vi "controlAutoReset.vi"(7 "Set":bool, 8 "error in":errorcluster, 9 "auto reset in":bool=TRUE, 10 "axis in":u8, 11 "connection ID":i32) -> (0 "error out":errorcluster, 1 "auto reset out":bool=TRUE, 2 "axis out":u8, 3 "connection ID":i32)   [LabVIEW 2016]
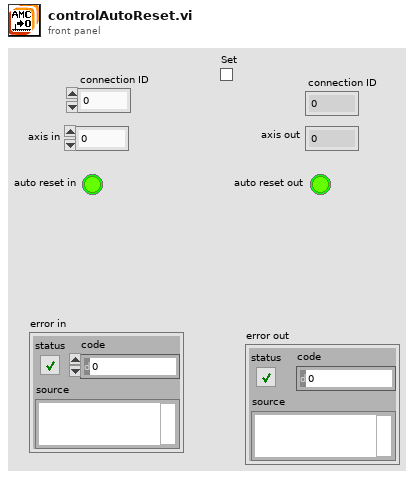
[diagram p1: front panel]
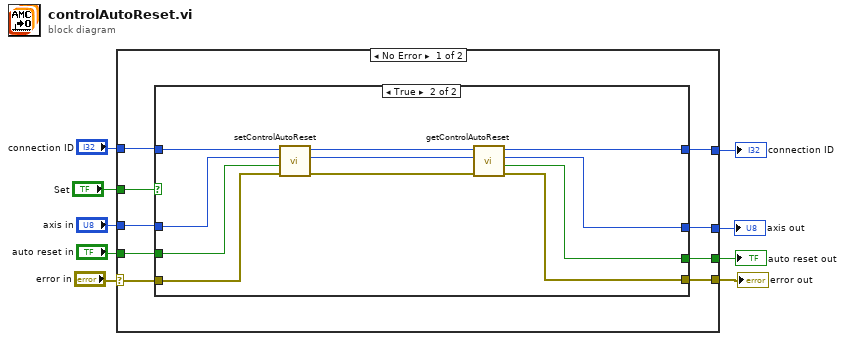
[diagram p0: block diagram]
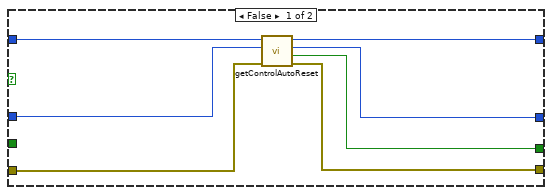
[diagram p2: hidden frame]
diagram:
  n1 = case shown="No Error" "error in" {
    selector: "error in" -> [w10 w40]
    tunnel: "axis in" -> [w16 w38]
    tunnel: [w11 w40] -> w8
    tunnel: [w13 w38] -> w7
    tunnel: "Set" -> [w17 _]
    tunnel: [w12 w39] -> w5
    tunnel: "auto reset in" -> [w15 w39]
    tunnel: [w14 w37] -> w1
    tunnel: "connection ID" -> [w18 w37]
    frame No Error {
      n2 = case shown="True" w17 {
        tunnel: [w24 w30] -> w14
        tunnel: w18 -> [w25 w36]
        tunnel: w16 -> [w19 w34]
        tunnel: [w21 w27] -> w13
        tunnel: [w20 w28] -> w12
        tunnel: [w22 w29] -> w11
        tunnel: w15 -> [_ w33]
        tunnel: w10 -> [w23 w35]
        frame False {
          n3 = call "getControlAutoReset.vi"("error in"=w23, "axis"=w19, "connection ID"=w25) -> ("error out"=w22:errorcluster, "enabled"=w20:bool, "axis_out"=w21:i32, "connection ID"=w24:i32)  [unwired: 5 in]
        }
        frame True {
          n4 = call "setControlAutoReset.vi"("error in"=w35, "enable"=w33, "axis"=w34, "connection ID"=w36) -> ("error out"=w32:errorcluster, "axis_out"=w26:i32, "connection ID"=w31:i32)  [unwired: 5 in]
          n5 = call "getControlAutoReset.vi"("error in"=w32, "axis"=w26, "connection ID"=w31) -> ("error out"=w29:errorcluster, "enabled"=w28:bool, "axis_out"=w27:i32, "connection ID"=w30:i32)  [unwired: 5 in]
        }
      }
    }
    frame Error {
    }
  }
  "error out" <- w8
  "axis out" <- w7
  "auto reset out" <- w5
  "connection ID" <- w1
